vi "TypesOfPIDControllers.vi"   [LabVIEW 2010]
uses:
  <vilib>/addons/control/pid/pid.llb/PID (DBL).vi
  <vilib>/addons/control/pid/pid.llb/PID Advanced (DBL).vi
  <vilib>/addons/control/pid/NI_PID_pid.lvlib
  <vilib>/addons/control/pid/NI_PID_autopid.lvlib
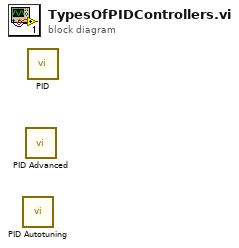
[diagram p0: block diagram]
diagram:
  n1 = call <vilib>:"PID Autotuning.vi"() -> ()  [unwired: 8 in, 4 out]
  n2 = call-poly <vilib>:"PID Advanced.vi"() -> ()  [unwired: 14 in, 2 out]
  n3 = call-poly <vilib>:"PID.vi"() -> ()  [unwired: 10 in, 2 out]
